vi "visionColor.vi"(3 "error in":errorcluster, 4 "Color":string="Default") -> (0 "error out":errorcluster, 1 "target position":i32, 2 "Array":u32[](array[colorbox]))   [LabVIEW 2019]
panel:
  out "original":T1(plugin-control)
  out "Image Out":T1(plugin-control)
  in  "Stop (F)":bool
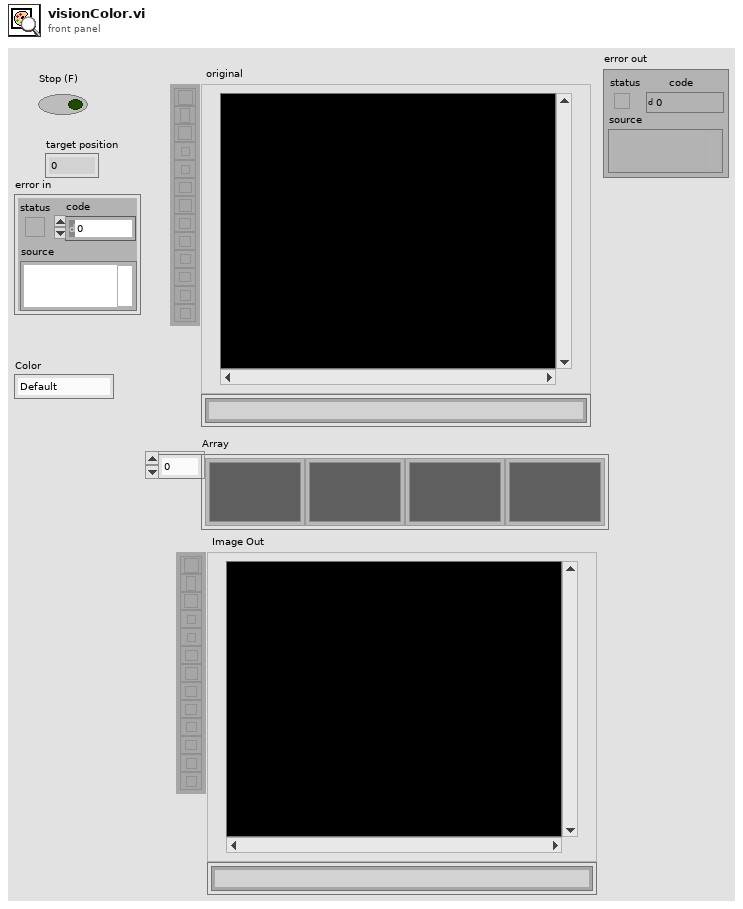
[diagram p1: front panel]
types:
  T1 = typedef "IMAQ Image.ctl" = refnum<image>
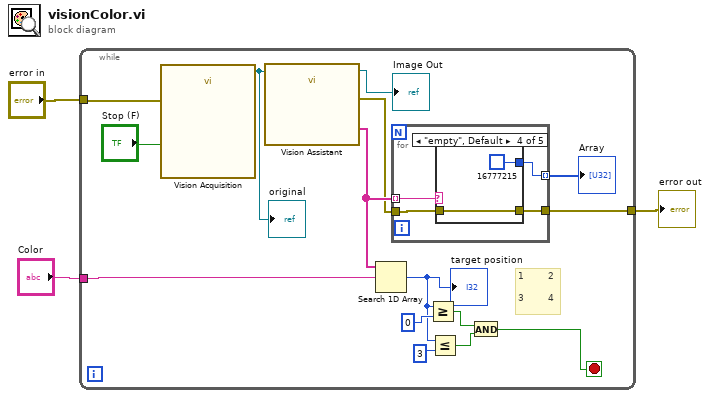
[diagram p0: block diagram]
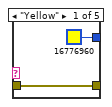
[diagram p2: hidden frame]
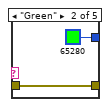
[diagram p3: hidden frame]
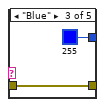
[diagram p4: hidden frame]
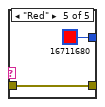
[diagram p5: hidden frame]
diagram:
  n1 = while {
    tunnel: "error in" -> [w11]
    tunnel: "Color" -> [w15]
    tunnel: [w13] -> w1
    stop <- w4 stop-if-true
    # "1        2\n\n3        4"
    n2 = call "Vision Acquisition"("Stop (F)"="Stop (F)", "error in"=w11) -> ("Image Out"=w10:T1)  [unwired: 23 in, 2 out]
    "original" <- w10
    n3 = call "Vision Assistant"("Image In"=w10) -> ("Image Out"=→"Image Out":T1, "Classes (Color Classification 1)"=w16:string[], "error out"=w14:errorcluster)  [unwired: 24 in]
    n4 = Search 1D Array(1D array=w16, element=w15) -> (index of element=w7:i32)  [unwired: 1 in]
    "target position" <- w7
    n5 = for {
      tunnel: [w22] -> w17 mode=indexing
      tunnel: w16 -> [w21] mode=indexing
      tunnel: w14 -> [w20]
      tunnel: [w19] -> w13
      n6 = case shown="\"empty\", Default" w21 {
        tunnel: [u32 16776960 u32 65280 u32 255 u32 16777215 u32 16711680] -> w22
        tunnel: [w23 w25 w27 w29 w31] -> w19
        tunnel: w20 -> [w23 w25 w27 w29 w31]
        frame "Yellow" {
        }
        frame "Green" {
        }
        frame "Blue" {
        }
        frame "empty", Default {
        }
        frame "Red" {
        }
      }
    }
    "Array" <- w17
    n7 = Greater Or Equal?(x=w7, y=0) -> (x >= y?=w6:bool)
    n8 = Less Or Equal?(x=w7, y=3) -> (x <= y?=w5:bool)
    n9 = And(x=w6, y=w5) -> (x .and. y?=w4:bool)
  }
  "error out" <- w1
